vi "Abort.vi"(8 "error in (no error)":errorcluster, 11 "ChromaPowerSupply in":refnum<class "ChromaPowerSupply.lvclass">) -> (0 "error out":errorcluster, 3 "ChromaPowerSupply out":refnum<class "ChromaPowerSupply.lvclass">)   [LabVIEW 2018, in "AcPwrPlugins.lvlib" / "ChromaPowerSupply.lvclass"]
uses:
  ChromaPowerSupply.lvclass
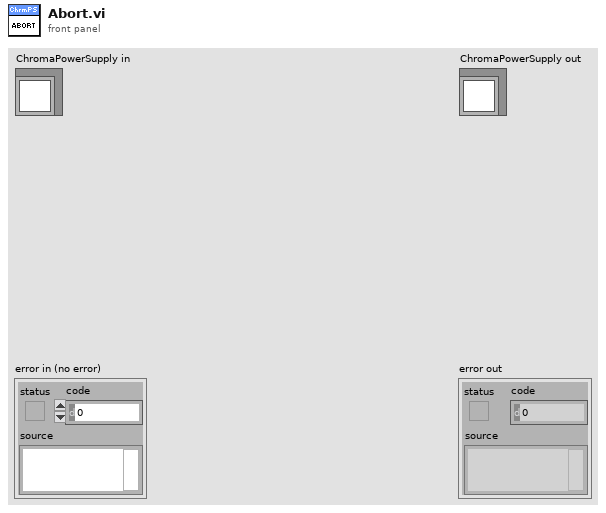
[diagram p1: front panel]
types:
  T1 = typedef "AcPwrPlugins.lvlib/ChromaPowerSupply.lvclass/Device(s)Settings.ctl" = cluster{"Phases":cluster{"Handle":string, "Instrument Options":string, "id query (T)":bool, "reset device (T)":bool, "Timing":cluster{"TimingOn":enum16{""}, "Hours":u32, "Minutes":u32, "Seconds":dbl, "CutoffVoltage":dbl}, "Connected":bool, "Output Mode":enum16{"Voltage (DC)", "Current (DC)"}, "Voltage":dbl, "Current":dbl, "Voltage Limit":dbl, "Current Limit":dbl}[], "MeasName":string}
  T2 = cluster{"Handle":string, "Instrument Options":string, "id query (T)":bool, "reset device (T)":bool, "Timing":cluster{"TimingOn":enum16{""}, "Hours":u32, "Minutes":u32, "Seconds":dbl, "CutoffVoltage":dbl}, "Connected":bool, "Output Mode":enum16{"Voltage (DC)", "Current (DC)"}, "Voltage":dbl, "Current":dbl, "Voltage Limit":dbl, "Current Limit":dbl}[]
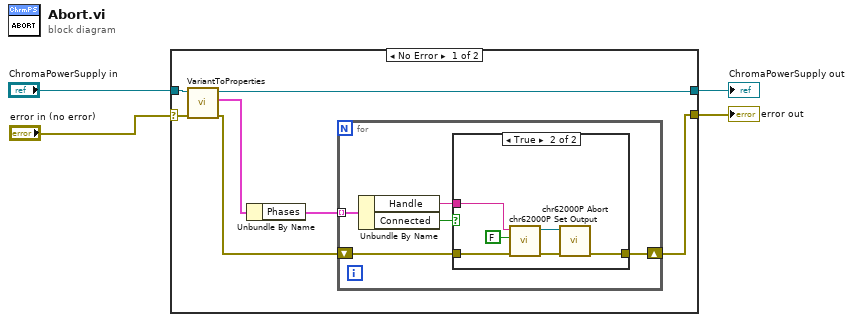
[diagram p0: block diagram]
diagram:
  n1 = case shown="No Error" "error in (no error)" {
    selector: "error in (no error)" -> [w10 w24]
    tunnel: [w7 w25] -> w3
    tunnel: "ChromaPowerSupply in" -> [w11 w25]
    tunnel: [w8 w24] -> w2
    frame No Error {
      n2 = call-dynamic "VariantToProperties.vi"("error in (no error)"=w10, "ChromaPowerSupply in"=w11) -> ("error out"=w9:errorcluster, "Device Settings"=w6:T1, "ChromaPowerSupply out"=w7:refnum<class "ChromaPowerSupply.lvclass">)  [unwired: 5 in, 2 out]
      n3 = Unbundle By Name(w6) -> ("Phases"=w5:T2)
      n4 = for {
        tunnel: w5 -> [w16] mode=indexing
        shift-right: [w14] -> w8
        shift-left: w9 -> [w15]
        n5 = Unbundle By Name(w16) -> ("Handle"=w13:string, "Connected"=w12:bool)
        n6 = case shown="True" w12 {
          tunnel: w13 -> [_ w20]
          tunnel: w15 -> [w17 w22]
          tunnel: [w17 w23] -> w14
          frame False {
          }
          frame True {
            n7 = call <instrlib>:"chr62000P Set Output.vi"("error in (no error)"=w22, "Output (Off)"=FALSE, "instrument handle"=w20) -> ("error out"=w21:errorcluster, "instrument handle out"=w19:refnum<k15>)  [unwired: 7 in]
            n8 = call <instrlib>:"chr62000P Abort.vi"("error in (no error)"=w21, "instrument handle"=w19) -> ("error out"=w23:errorcluster)  [unwired: 8 in, 1 out]
          }
        }
      }
    }
    frame Error {
    }
  }
  "error out" <- w2
  "ChromaPowerSupply out" <- w3
